vi "AgeInYears.vi"(2 "Birthday":timestamp, 3 "Current Date":timestamp) -> (0 "?":string, 1 "Age (Years)":i16)   [LabVIEW 2020]
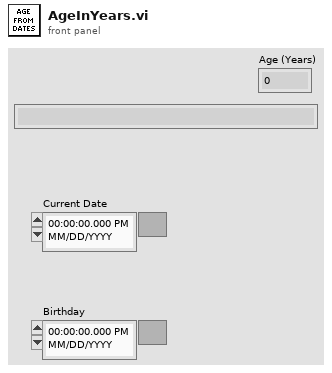
[diagram p1: front panel]
types:
  T1 = typedef "LVDateTimeRec.ctl" = cluster{"fractional second":dbl, "second":i32, "minute":i32, "hour":i32, "day of month":i32, "month":i32, "year":i32, "day of week":i32, "day of year":i32, "DST":i32}
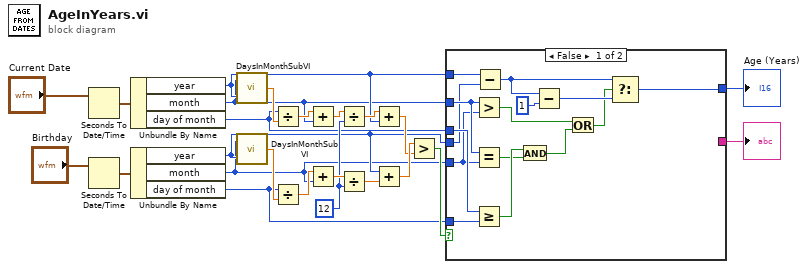
[diagram p0: block diagram]
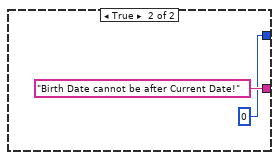
[diagram p2: hidden frame]
diagram:
  w18 = 12
  n1 = Seconds To Date/Time(time stamp (now)="Current Date") -> (date time rec=w4:T1)  [unwired: 1 in]
  n2 = Seconds To Date/Time(time stamp (now)="Birthday") -> (date time rec=w9:T1)  [unwired: 1 in]
  n3 = Unbundle By Name(w4) -> ("year"=w3:i32, "month"=w2:i32, "day of month"=w1:i32)
  n4 = Unbundle By Name(w9) -> ("year"=w8:i32, "month"=w7:i32, "day of month"=w6:i32)
  n5 = call "DaysInMonthSubVI.vi"("Year"=w3, "Month"=w2) -> ("Max Days in Month"=w24:dbl)
  n6 = call "DaysInMonthSubVI.vi"("Year"=w8, "Month"=w7) -> ("Max Days in Month"=w23:dbl)
  n7 = Divide(x=w1, y=w24) -> (x/y=w22:dbl)
  n8 = Divide(x=w6, y=w23) -> (x/y=w21:dbl)
  n9 = Add(x=w22, y=w2) -> (x+y=w20:dbl)
  n10 = Add(x=w21, y=w7) -> (x+y=w19:dbl)
  n11 = Divide(x=w20, y=w18) -> (x/y=w17:dbl)
  n12 = Divide(x=w19, y=w18) -> (x/y=w16:dbl)
  n13 = Add(x=w17, y=w3) -> (x+y=w14:dbl)
  n14 = Add(x=w8, y=w16) -> (x+y=w15:dbl)
  n15 = Greater?(x=w15, y=w14) -> (0:w13:bool)
  n16 = case shown="False" w13 {
    tunnel: [_ "Birth Date cannot be after Current Date!"] -> w12
    tunnel: [w39 0] -> w11
    tunnel: w2 -> [w35 _]
    tunnel: w7 -> [w33 _]
    tunnel: w1 -> [w34 _]
    tunnel: w3 -> [w28 _]
    tunnel: w8 -> [w27 _]
    tunnel: w6 -> [w25 _]
    frame False {
      n17 = Greater?(x=w35, y=w33) -> (0:w36:bool)
      n18 = Equal?(x=w35, y=w33) -> (x = y?=w31:bool)
      n19 = Greater Or Equal?(x=w34, y=w25) -> (x >= y?=w32:bool)
      n20 = Subtract(x=w28, y=w27) -> (x-y=w26:i32)
      n21 = And(x=w32, y=w31) -> (x .and. y?=w30:bool)
      n22 = Subtract(x=w26, y=1) -> (x-y=w37:i32)
      n23 = Or(x=w36, y=w30) -> (x .or. y?=w29:bool)
      n24 = Select(t=w26, s=w29, f=w37) -> (s? t:f=w39:i32)
    }
    frame True {
    }
  }
  "Age (Years)" <- w11
  "?" <- w12
